vi "call_python_node.vi"() -> ()   [LabVIEW 2019]
panel:
  out "error out":errorcluster
  out "session out":refnum<k35>
  in  "error in (no error)":errorcluster
  in  "function name":string
  in  "module path":path
  in  "session in":refnum<k35>
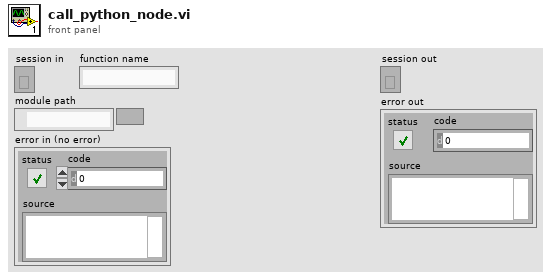
[diagram p1: front panel]
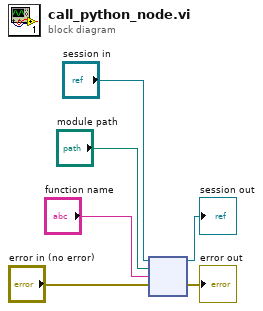
[diagram p0: block diagram]
diagram:
  n1 = node("session in", "module path", "function name", "error in (no error)") -> (→"session out":refnum<k35>, →"error out":errorcluster)  [unwired: 2 in, 2 out]
